vi "Vision Processing.vi"(4 "error in (no error)":errorcluster, 7 "Image Size":T1=enum."320x240") -> ()   [LabVIEW 2016]
doc: "This VI runs in parallel to other tasks. It gets images from the camera, processes them for color or shape and uses commands or globals to affect the behavior of other subsystems."
uses:
  <vilib>/Rock Robotics/WPI/Camera/WPI_CameraImageSize.ctl
  <vilib>/Rock Robotics/WPI/Camera/WPI_CameraWhite Balance Values.ctl
  <vilib>/Rock Robotics/WPI/Camera/WPI_CameraExposure Values.ctl
  <vilib>/Rock Robotics/WPI/Camera/WPI_CameraFrameRate.ctl
  Framework/Robot Global Data.vi
panel:
  in  "Image Size 2":T1=enum."320x240"
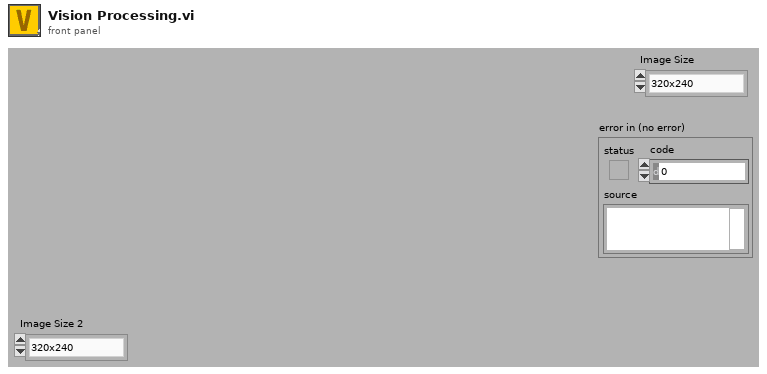
[diagram p1: front panel]
types:
  T1 = typedef "WPI_CameraImageSize.ctl" = enum16{"640x480", "320x240", "160x120", "Custom"}
  T2 = typedef "WPI_CameraFrameRate.ctl" = u32
  T3 = typedef "WPI_CameraExposure Values.ctl" = enum16{"Auto", "Flicker-free 50 Hz", "Flicker-free 60 Hz", "Hold current", "Custom"}
  T4 = typedef "WPI_CameraWhite Balance Values.ctl" = enum16{"Auto", "Fixed indoor", "Fixed outdoor 1", "Fixed outdoor 2", "Fixed fluorescent 1", "Fixed fluorescent 2", "Hold current", "Custom"}
  T5 = typedef "Image Type" = u32
  T6 = typedef "WPI_CameraDevRef.ctl" = cluster{"Camera Address":string, "CameraStatus":errorcluster}
  T7 = typedef "IMAQ Image.ctl" = refnum<image>
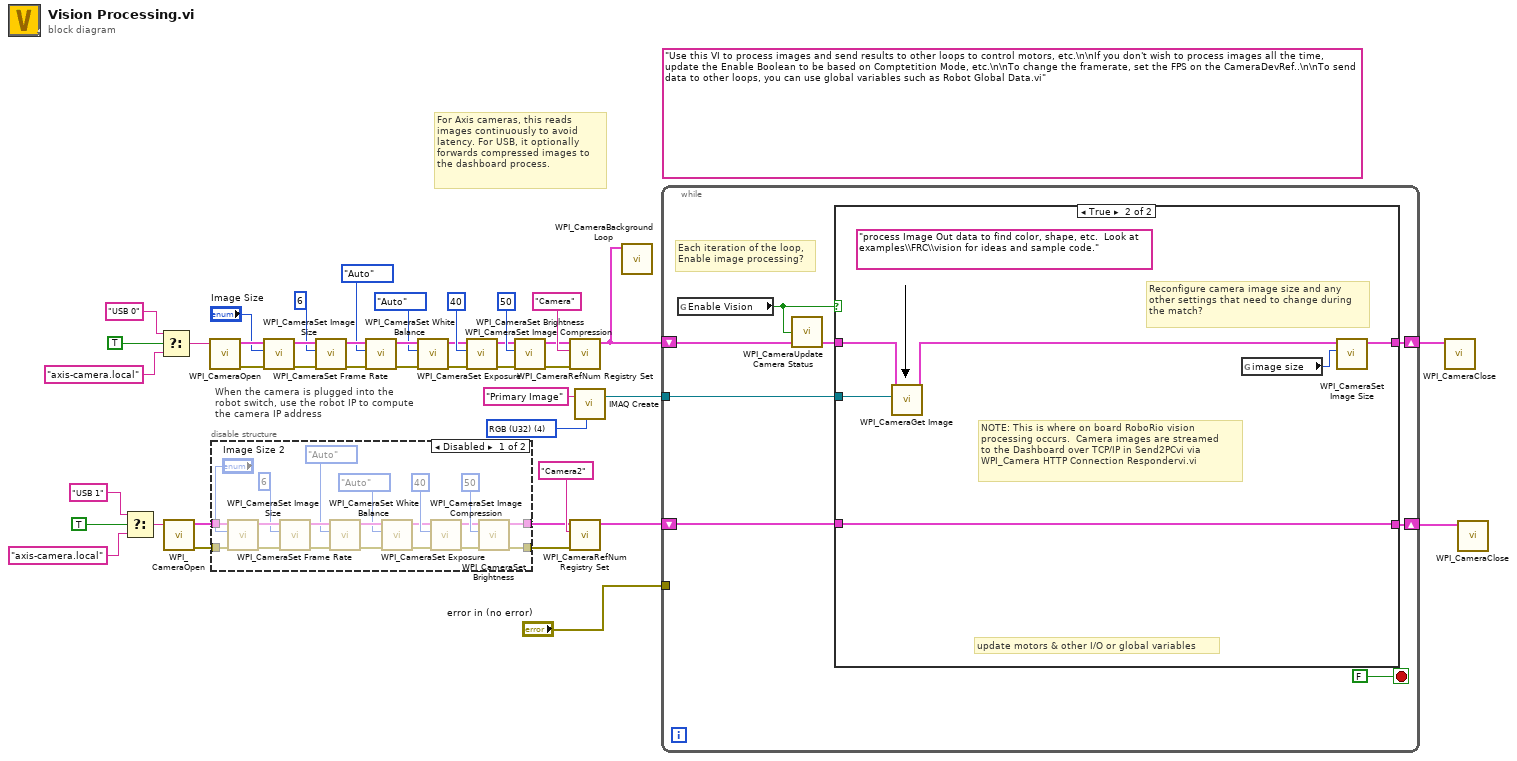
[diagram p0: block diagram]
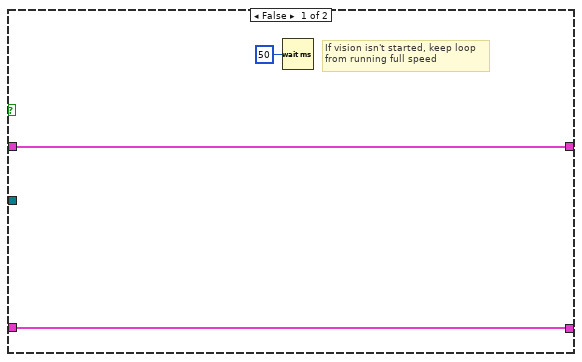
[diagram p3: hidden frame]
diagram:
  (unwired) "Use this VI to process images and send results to other loops to control motors, etc.\n\nIf you don't wish to process images all the time, update the Enable Boolean to be based on Comptetition Mode, etc.\n\nTo change the framerate, set the FPS on the CameraDevRef..\n\nTo send data to other loops, you can use global variables such as Robot Global Data.vi"
  w42 = T5 4 items=["Grayscale (U8)", "Grayscale (I16)", "Grayscale (SGL)", "Complex (CSG)", "RGB (U32)", "HSL (U32)", "RGB (U64)"] ("Image Type")
  # "When the camera is plugged into the\nrobot switch, use the robot IP to compute\nthe camera IP address"
  # "For Axis cameras, this reads\nimages continuously to avoid\nlatency. For USB, it optionally\nforwards compressed images to\nthe dashboard process."
  n1 = Select(t="USB 1" ("format string"), s=TRUE ("dot notation? (F)"), f="axis-camera.local" ("format string")) -> (s? t:f=w4:string)
  n2 = Select(t="USB 0" ("format string"), s=TRUE ("dot notation? (F)"), f="axis-camera.local" ("format string")) -> (s? t:f=w13:string)
  n3 = call <vilib>:"WPI_CameraOpen.vi"("Camera Address"=w4) -> ("error out"=w9:errorcluster, "CameraDevRef"=w10:T6)  [unwired: 1 in, 8 out]
  n4 = call <vilib>:"WPI_CameraOpen.vi"("Camera Address"=w13) -> ("error out"=w30:errorcluster, "CameraDevRef"=w31:T6)  [unwired: 1 in, 8 out]
  n5 = disable-structure shown="Disabled" {
    disable-tunnel: w10 -> [w55 w63]
    disable-tunnel: w9 -> [w54 w64]
    disable-tunnel: [w48 w63] -> w8
    disable-tunnel: [w47 w64] -> w7
    frame Disabled {
      n6 = call <vilib>:"WPI_CameraSet Image Size.vi"("error in (no error)"=w54, "Image Size"="Image Size 2", "CameraDevRef"=w55) -> ("error out"=w53:errorcluster, "CameraDevRef Out"=w56:T6)  [unwired: 1 in, 6 out]
      n7 = call <vilib>:"WPI_CameraSet Frame Rate.vi"("error in (no error)"=w53, "Frame Rate (fps)"=T2 6, "CameraDevRef"=w56) -> ("error out"=w52:errorcluster, "CameraDevRef Out"=w58:T6)  [unwired: 7 out]
      n8 = call <vilib>:"WPI_CameraSet White Balance.vi"("error in (no error)"=w52, "White Balance"=WPI_CameraWhite_Balance_Values."Auto", "CameraDevRef"=w58) -> ("error out"=w51:errorcluster, "CameraDevRef Out"=w57:T6)  [unwired: 1 in, 6 out]
      n9 = call <vilib>:"WPI_CameraSet Exposure.vi"("error in (no error)"=w51, "Exposure"=WPI_CameraExposure_Values."Auto", "CameraDevRef"=w57) -> ("error out"=w50:errorcluster, "CameraDevRef Out"=w60:T6)  [unwired: 1 in, 6 out]
      n10 = call <vilib>:"WPI_CameraSet Image Compression.vi"("error in (no error)"=w50, "Compression"=40, "CameraDevRef"=w60) -> ("error out"=w49:errorcluster, "CameraDevRef Out"=w59:T6)  [unwired: 7 out]
      n11 = call <vilib>:"WPI_CameraSet Brightness.vi"("error in (no error)"=w49, "Brightness"=50, "CameraDevRef"=w59) -> ("error out"=w47:errorcluster, "CameraDevRef Out"=w48:T6)  [unwired: 7 out]
    }
    frame Enabled {
    }
  }
  n12 = call <vilib>:"WPI_CameraSet Image Size.vi"("error in (no error)"=w30, "Image Size"="Image Size", "CameraDevRef"=w31) -> ("error out"=w29:errorcluster, "CameraDevRef Out"=w32:T6)  [unwired: 1 in, 6 out]
  n13 = call <vilib>:"WPI_CameraSet Frame Rate.vi"("error in (no error)"=w29, "Frame Rate (fps)"=T2 6, "CameraDevRef"=w32) -> ("error out"=w28:errorcluster, "CameraDevRef Out"=w34:T6)  [unwired: 7 out]
  n14 = call <vilib>:"WPI_CameraSet White Balance.vi"("error in (no error)"=w28, "White Balance"=WPI_CameraWhite_Balance_Values."Auto", "CameraDevRef"=w34) -> ("error out"=w27:errorcluster, "CameraDevRef Out"=w33:T6)  [unwired: 1 in, 6 out]
  n15 = call <vilib>:"WPI_CameraSet Exposure.vi"("error in (no error)"=w27, "Exposure"=WPI_CameraExposure_Values."Auto", "CameraDevRef"=w33) -> ("error out"=w26:errorcluster, "CameraDevRef Out"=w36:T6)  [unwired: 1 in, 6 out]
  n16 = call <vilib>:"WPI_CameraSet Image Compression.vi"("error in (no error)"=w26, "Compression"=40, "CameraDevRef"=w36) -> ("error out"=w25:errorcluster, "CameraDevRef Out"=w35:T6)  [unwired: 7 out]
  n17 = call <vilib>:"WPI_CameraSet Brightness.vi"("error in (no error)"=w25, "Brightness"=50, "CameraDevRef"=w35) -> ("error out"=w23:errorcluster, "CameraDevRef Out"=w24:T6)  [unwired: 7 out]
  n18 = call <vilib>:"WPI_CameraRefNum Registry Set.vi"("error in (no error)"=w23, "refnum name"="Camera", "CameraDevRef"=w24) -> ("CameraDevRef"=w19:T6)  [unwired: 1 in, 7 out]
  n19 = call <vilib>:"WPI_CameraRefNum Registry Set.vi"("error in (no error)"=w7, "refnum name"="Camera2", "CameraDevRef"=w8) -> ("CameraDevRef"=w2:T6)  [unwired: 1 in, 7 out]
  n20 = call "IMAQ Create"("Image Name"="Primary Image", "Image Type"=w42) -> ("New Image"=w40:T7)  [unwired: 2 in, 2 out]
  n21 = call <vilib>:"WPI_CameraBackground Loop.vi"("CameraDevRef"=w19) -> ()  [unwired: 11 in]
  n22 = while {
    shift-right: [w71] -> w17
    shift-left: w19 -> [w69]
    tunnel: w40 -> [w70]
    tunnel: "error in (no error)" -> [_]
    shift-right: [w65] -> w1
    shift-left: w2 -> [w66]
    stop <- FALSE stop-if-true
    # "Each iteration of the loop,\nEnable image processing?"
    n23 = global read "Robot Global Data.vi" "Enable Vision"() -> (w67:bool)
    n24 = call <vilib>:"WPI_CameraUpdate Camera Status.vi"("CameraDevRef In"=w69, "Enable Vision"=w67) -> ("CameraDevRef Out"=w68:T6)  [unwired: 3 in]
    n25 = case shown="True" w67 {
      tunnel: w70 -> [_ w80]
      tunnel: [w75 w81] -> w71
      tunnel: w68 -> [w75 w78]
      tunnel: w66 -> [w73 w76]
      tunnel: [w73 w76] -> w65
      frame False {
        # "If vision isn't started, keep loop\nfrom running full speed"
        n26 = Wait (ms)(milliseconds to wait=u32 50) -> ()  [unwired: 1 out]
      }
      frame True {
        (unwired) "process Image Out data to find color, shape, etc.  Look at examples\\FRC\\vision for ideas and sample code."
        # "NOTE: This is where on board RoboRio vision\nprocessing occurs.  Camera images are streamed \nto the Dashboard over TCP/IP in Send2PCvi via\nWPI_Camera HTTP Connection Respondervi.vi"
        # "update motors & other I/O or global variables"
        # "Reconfigure camera image size and any\nother settings that need to change during\nthe match?"
        n27 = call <vilib>:"WPI_CameraGet Image.vi"("Image"=w80, "CameraDevRef"=w78) -> ("CameraDevRef Out"=w77:T6)  [unwired: 1 in, 8 out]
        n28 = global read "Robot Global Data.vi" "image size"() -> (w79:T1)
        n29 = call <vilib>:"WPI_CameraSet Image Size.vi"("Image Size"=w79, "CameraDevRef"=w77) -> ("CameraDevRef Out"=w81:T6)  [unwired: 2 in, 7 out]
      }
    }
  }
  n30 = call <vilib>:"WPI_CameraClose.vi"("CameraDevRef"=w17) -> ()  [unwired: 1 in, 10 out]
  n31 = call <vilib>:"WPI_CameraClose.vi"("CameraDevRef"=w1) -> ()  [unwired: 1 in, 10 out]
